vi "load_hardware_from_absolute_path.vi"(8 "error in (no error)":errorcluster, 11 "absolute path":path) -> (0 "error out":errorcluster, 3 "Hardware out":refnum<class "Hardware.lvclass">)   [LabVIEW 2017, in "Hardware.lvclass"]
doc: "Load the hardware from an absolute path"
uses:
  Hardware.lvclass
  <vilib>/Utility/error.llb/Error Cluster From Error Code.vi
  <vilib>/ErrorRing/Error Ring.xnode
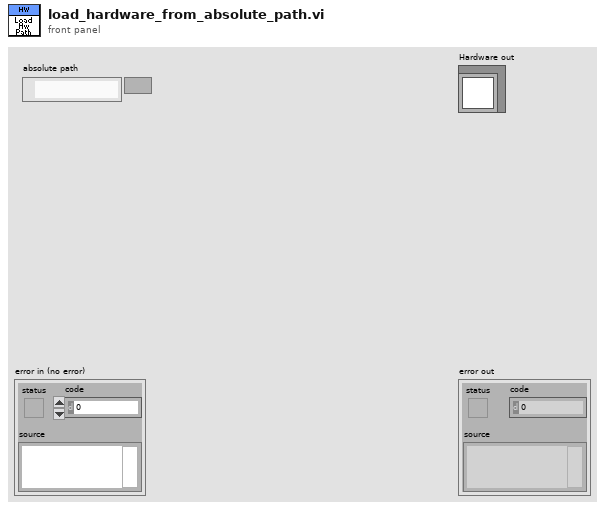
[diagram p1: front panel]
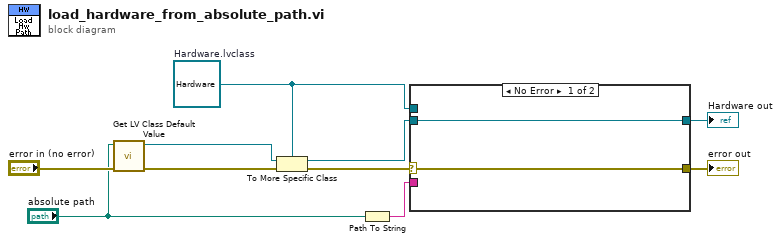
[diagram p0: block diagram]
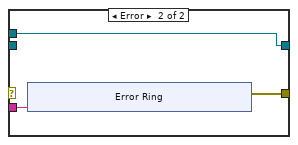
[diagram p2: hidden frame]
diagram:
  w4 = refnum<class "Hardware.lvclass"> refnum  # Hardware.lvclass
  n1 = call <vilib>:"Get LV Class Default Value.vi"("error in (no error)"="error in (no error)", "class path"="absolute path") -> ("error out"=w8:errorcluster, "object"=w9:refnum<class>)  [unwired: 8 in]
  n2 = To More Specific Class(target class=w4, reference=w9, error in=w8) -> (specific class reference=w6:refnum<class "Hardware.lvclass">, error out=w7:errorcluster)
  n3 = Path To String(path="absolute path") -> (string=w1:string)
  n4 = case shown="No Error" w7 {
    selector: w7 -> [w11 _]
    tunnel: w6 -> [w12 _]
    tunnel: [w12 w15] -> w5
    tunnel: w4 -> [_ w15]
    tunnel: [w11 w14] -> w3
    tunnel: w1 -> [_ w13]
    frame No Error {
    }
    frame Error {
      n5 = xnode "Error Ring"("parameter 0"=w13) -> ("error out"=w14:errorcluster)
    }
  }
  "error out" <- w3
  "Hardware out" <- w5
